vi "DMA.Write Block.vi"(8 "error in (no error)":errorcluster, 9 "data":dbl[](array[numeric]), 10 "block index":i32, 11 "GE 5565 params":T1 {"DMA Blocks"."size" format="%08x"; "DMA Blocks"."pointer" format="%08x"}) -> (0 "error out":errorcluster, 2 "block index out":i32, 3 "GE 5565 params out":T1 {"DMA Blocks"."size" format="%08x"; "DMA Blocks"."pointer" format="%08x"})   [LabVIEW 2016, in "GE 5565PIORC.lvclass"]
uses:
  GE 5565PIORC.lvclass
  Controls/GE 5565 Params.ctl
  Controls/DMA Block.ctl
  Controls/DMA Config.ctl
  <vilib>/Instr/_visa.llb/VISA Register Access Address Space.ctl
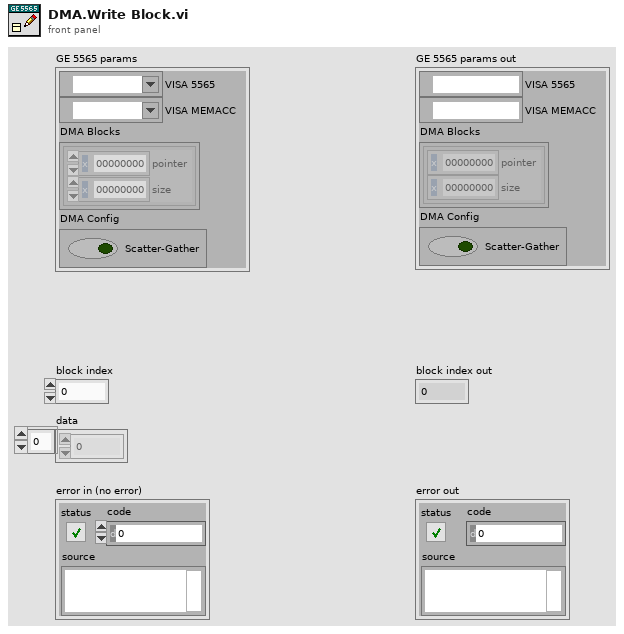
[diagram p1: front panel]
types:
  T1 = typedef "GE 5565PIORC.lvclass/GE 5565 Params.ctl" = cluster{"VISA 5565":refnum<visa-resource-name>, "VISA MEMACC":refnum<visa-resource-name>, "DMA Blocks":T2[], "DMA Config":T3}
  T2 = typedef "GE 5565PIORC.lvclass/DMA Block.ctl" = cluster{"pointer":u32, "size":u32}
  T3 = typedef "GE 5565PIORC.lvclass/DMA Config.ctl" = cluster{"Scatter-Gather":bool}
  T4 = typedef "VISA Register Access Address Space.ctl" = u16
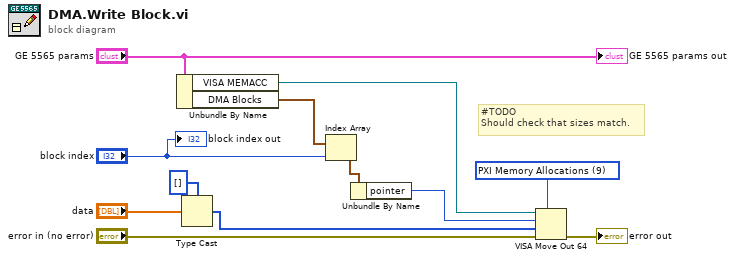
[diagram p0: block diagram]
diagram:
  w8 = T4 9 items=["VXI/VME A16"=1, "VXI/VME A24"=2, "VXI/VME A32"=3, "VXI/VME A64"=4, "PXI Memory Allocations"=9, "PXI Configuration"=10, "PXI BAR0"=11, "PXI BAR1"=12, "PXI BAR2"=13, "PXI BAR3"=14, "PXI BAR4"=15, "PXI BAR5"=16] ("Address Space")
  # "#TODO\nShould check that sizes match."
  n1 = Unbundle By Name("GE 5565 params") -> ("VISA MEMACC"=w3:refnum<visa-resource-name>, "DMA Blocks"=w2:T2[])
  n2 = Type Cast(type=u64[] [] ("initialized array"), x="data") -> (*(type *) &x=w10:u64[])
  n3 = Index Array(array=w2, index="block index") -> (element=w6:T2)
  n4 = Unbundle By Name(w6) -> ("pointer"=w7:u32)
  n5 = VISA Move Out 64(7:w8, 8:"error in (no error)", 9:w10, 10:w7, 11:w3) -> (0:→"error out":errorcluster)  [unwired: 1 out]
  "GE 5565 params out" <- "GE 5565 params"
  "block index out" <- "block index"
